vi "read_acq_mode.vi"(8 "error in (no error)":errorcluster, 11 "tt20 in":refnum<class "tt20.lvclass">) -> (0 "error out":errorcluster, 2 "Mode":T1 items=["T2"=2, "T3"=3], 3 "tt20 out":refnum<class "tt20.lvclass">)   [LabVIEW 2015, in "tt20.lvclass"]
uses:
  tt20.lvclass
  Picoquant/Hydraharp/hydraharp_panel/hpanel_acq_modes.ctl
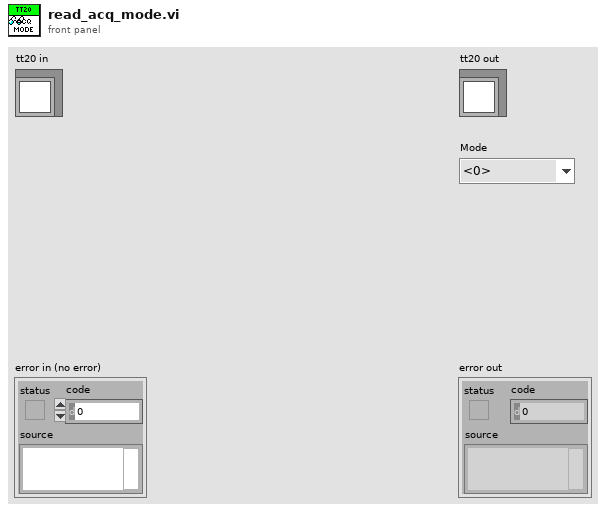
[diagram p1: front panel]
types:
  T1 = typedef "hpanel_acq_modes.ctl" = u16
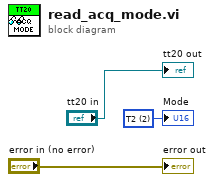
[diagram p0: block diagram]
diagram:
  w2 = T1 2 items=["T2"=2, "T3"=3] ("Mode")
  "error out" <- "error in (no error)"
  "tt20 out" <- "tt20 in"
  "Mode" <- w2
